vi "BME_DG_ReadParameterFile.vi"(8 "error in (no error)":errorcluster, 11 "Path":path=path "C:/Dokumente und Einstellungen/A2.5/Desktop/201203-22 Test mit vier DG.g0y") -> (0 "error out":errorcluster, 1 "Slave or Master":T1[](array[typedef]), 2 "DGs":T4, 3 "#DGs":i32, 4 "CalibrateTiming":u32, 5 "CalibrationLevel":u32)   [LabVIEW 2009]
uses:
  Typedefs For ReadParameters()/BME_DG_BME_State.ctl
  Typedefs For ReadParameters()/BME_DG_DelayChannelData.ctl
  BME_DG_MasterOrSlave.ctl
  BME Beispiele/BME DLL/DelayGenerator.dll
panel:
  in  "Cluster":T4
  in  "p_CalibrationLevel":u32
  in  "p_CalibrateTiming":u32
  in  "#DG in":i32
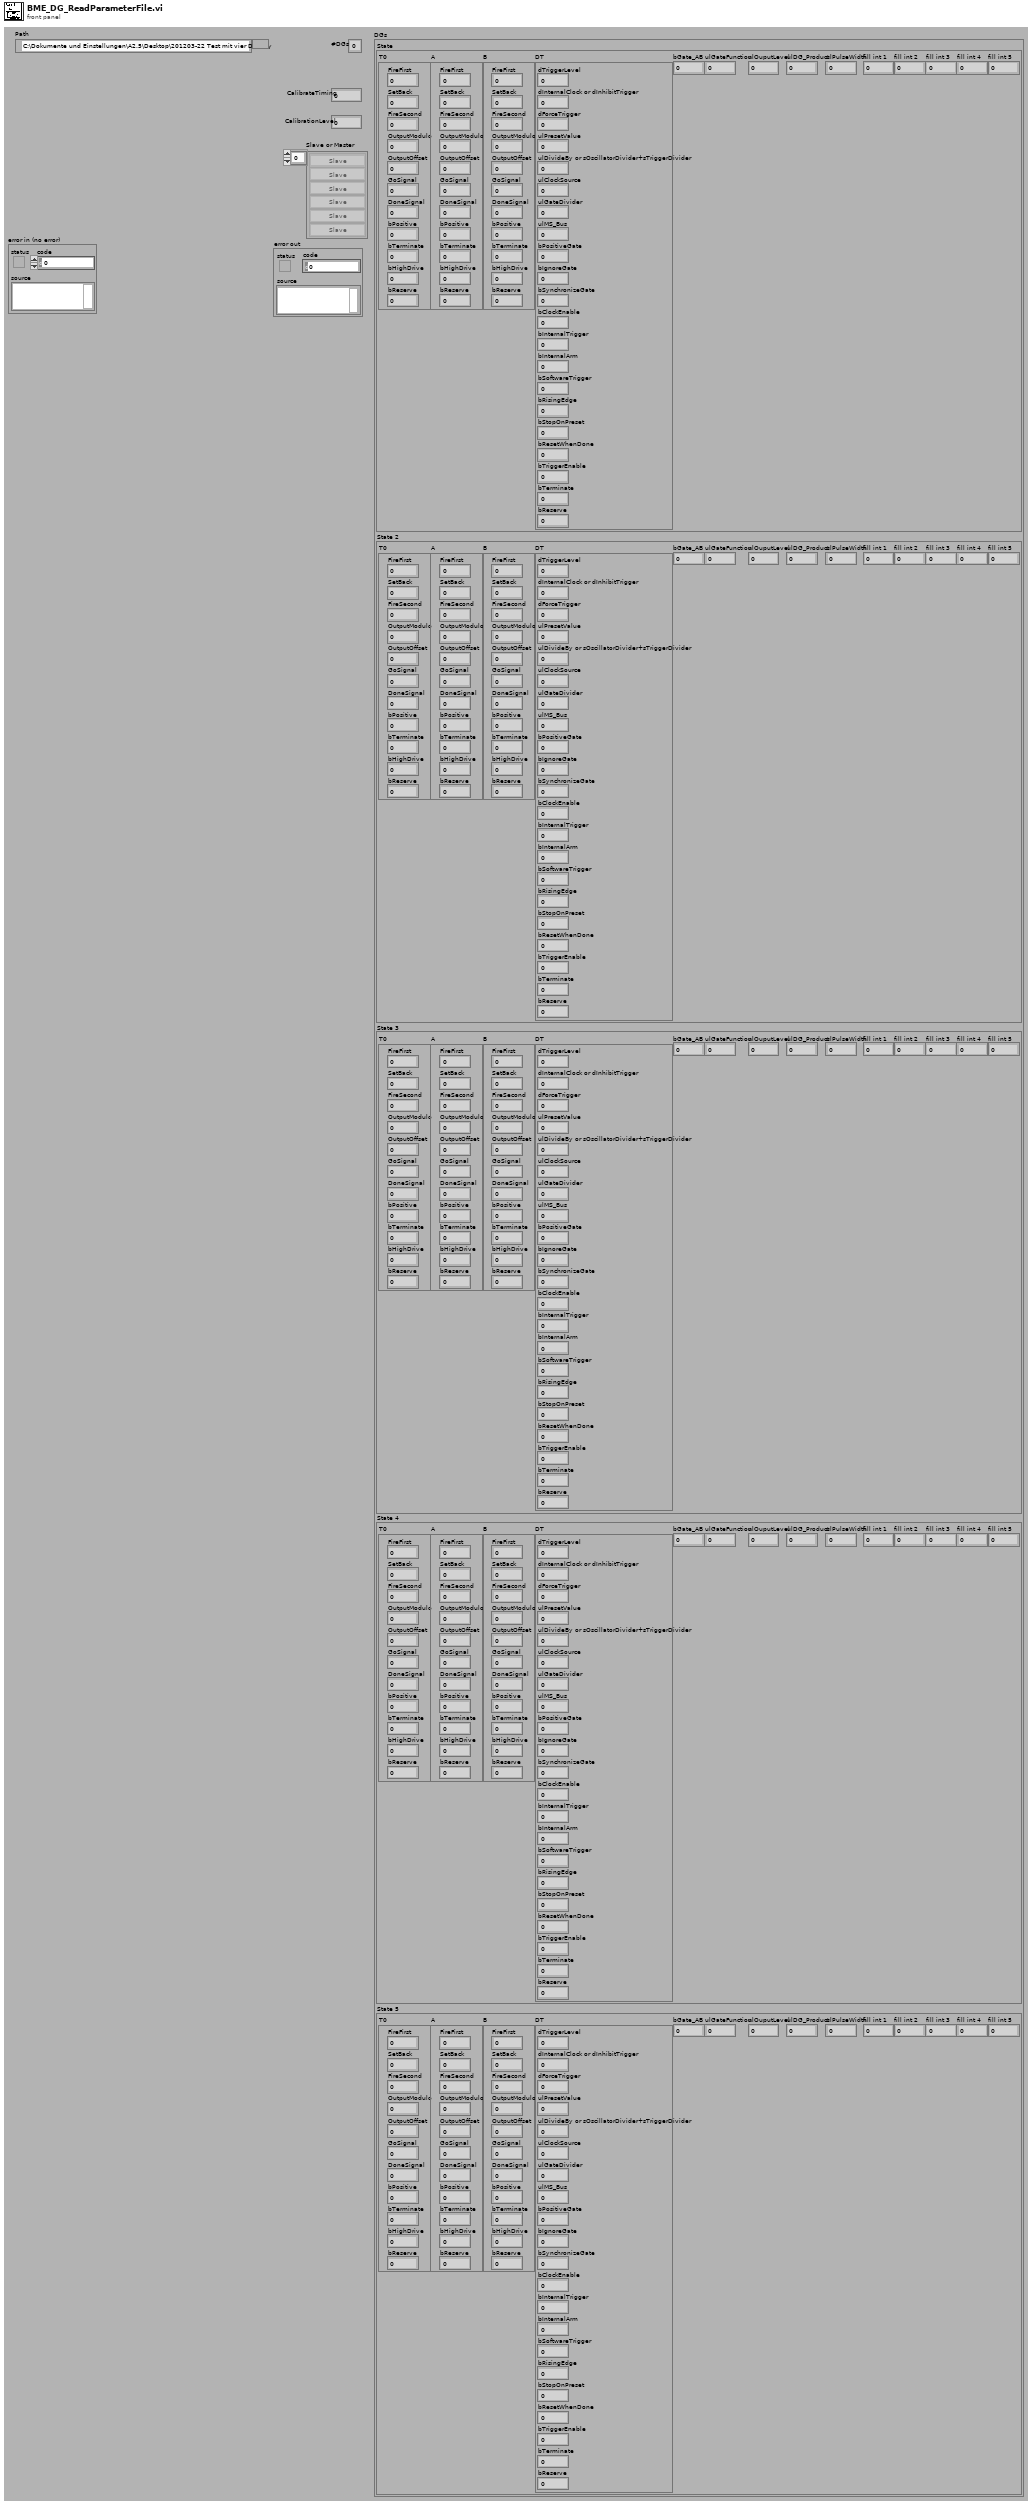
[diagram p1: front panel]
types:
  T1 = typedef "BME_DG_MasterOrSlave.ctl" = enum16{"Unknown", "Master", "Slave"}
  T2 = typedef "BME_DG_BME_State.ctl" = cluster{"T0":T3, "A":T3, "B":T3, "DT":cluster{"dTriggerLevel":dbl, "dInternalClock or dInhibitTrigger":dbl, "dForceTrigger":dbl, "ulPresetValue":u32, "ulDivideBy or sOscillatorDivider+sTriggerDivider":u32, "ulClockSource":u32, "ulGateDivider":u32, "ulMS_Bus":u32, "bPositiveGate":u32, "bIgnoreGate":u32, "bSynchronizeGate":u32, "bClockEnable":u32, "bInternalTrigger":u32, "bInternalArm":u32, "bSoftwareTrigger":u32, "bRisingEdge":u32, "bStopOnPreset":u32, "bResetWhenDone":u32, "bTriggerEnable":u32, "bTerminate":u32, "bReserve":u32}, "bGate_AB":u32, "ulGateFunction":u32, "ulOuputLevel":u32, "ulDG_Product":u32, "ulPulseWidth":u32, "fill int 1":i32, "fill int 2":i32, "fill int 3":i32, "fill int 4":i32, "fill int 5":i32}
  T3 = typedef "BME_DG_DelayChannelData.ctl" = cluster{"FireFirst":dbl, "SetBack":dbl, "FireSecond":dbl, "OutputModulo":u32, "OutputOffset":u32, "GoSignal":u32, "DoneSignal":u32, "bPositive":u32, "bTerminate":u32, "bHighDrive":u32, "bReserve":u32}
  T4 = cluster{"State":T2, "State 2":T2, "State 3":T2, "State 4":T2, "State 5":T2}
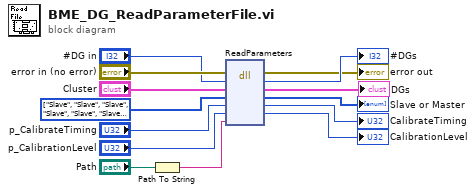
[diagram p0: block diagram]
diagram:
  w1 = T1[] [enum."Slave", enum."Slave", enum."Slave", enum."Slave", enum."Slave", enum."Slave", enum."Slave", enum."Slave", enum."Slave", enum."Slave", enum."Slave", enum."Slave", enum."Slave", enum."Slave", enum."Slave", enum."Slave", enum."Slave", enum."Slave", enum."Slave", enum."Slave", enum."Slave", enum."Slave", enum."Slave", enum."Slave", enum."Slave", enum."Slave", enum."Slave", enum."Slave", enum."Slave", enum."Slave", enum."Slave", enum."Slave", enum."Slave", enum."Slave", enum."Slave", enum."Slave", enum."Slave", enum."Slave", enum."Slave", enum."Slave", enum."Slave", enum."Slave", enum."Slave", enum."Slave", enum."Slave", enum."Slave", enum."Slave", enum."Slave", enum."Slave", enum."Slave", enum."Unknown"] items=["Unknown", "Master", "Slave"]
  n1 = Path To String(path="Path") -> (string=w9:string)
  n2 = dll-call lib="C:/Dokumente und Einstellungen/A2.5/Desktop/BME Beispiele/BME DLL/DelayGenerator.dll" fn="ReadParameters" label="Activate_DG_BME"(error in="error in (no error)", "#DG"="#DG in", "DGS"="Cluster", "module"=w1, "CalibrateTiming"="p_CalibrateTiming", "CalibrationLevel"="p_CalibrationLevel", "FileName"=w9) -> (error out=→"error out":errorcluster, "#DG"=→"#DGs":i32, "DGS"=→"DGs":T4, "module"=→"Slave or Master":i32[], "CalibrateTiming"=→"CalibrateTiming":u32, "CalibrationLevel"=→"CalibrationLevel":u32)  [unwired: 2 in, 1 out]
